vi "Create solenoid.vi"(7 "Variant":variant, 8 "error in (no error)":errorcluster, 9 "Reverse solenoid channel":string, 10 "Forward solenoid channel":string, 11 "Solenoids in":refnum<class "Solenoids.lvclass">) -> (0 "error out":errorcluster, 3 "Solenoids out":refnum<class "Solenoids.lvclass">)   [LabVIEW 2018, in "Pneumatics control.lvlib" / "Pneumatics.lvclass"]
doc: "This VI reads the string keys of the solenoid and sets them to the object using its Begin.vi"
uses:
  Pneumatics.lvclass
  Solenoids/Solenoids.lvclass
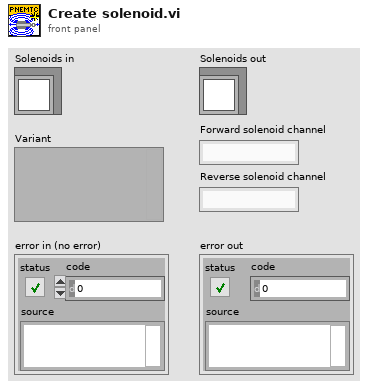
[diagram p1: front panel]
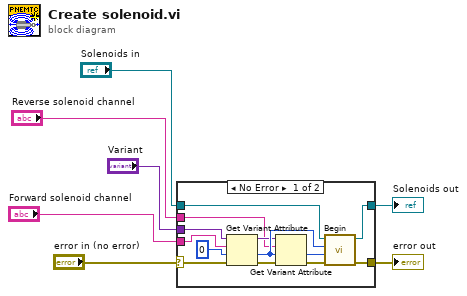
[diagram p0: block diagram]
diagram:
  n1 = case shown="No Error" "error in (no error)" {
    selector: "error in (no error)" -> [w12 w22]
    tunnel: [w19 w22] -> w7
    tunnel: "Variant" -> [w16 _]
    tunnel: "Solenoids in" -> [w11 w21]
    tunnel: [w10 w21] -> w3
    tunnel: "Forward solenoid channel" -> [w9 _]
    tunnel: "Reverse solenoid channel" -> [w8 _]
    frame No Error {
      n2 = Get Variant Attribute(Variant=w16, name=w9, default value (empty Variant)=u8 0, error in=w12) -> (duplicate Variant=w15:variant, value=w20:u8, error out=w13:errorcluster)  [unwired: 1 out]
      n3 = Get Variant Attribute(Variant=w15, name=w8, default value (empty Variant)=w20, error in=w13) -> (value=w18:u8, error out=w14:errorcluster)  [unwired: 2 out]
      n4 = call-dynamic "Begin.vi"("error in (no error)"=w14, "Reverse solenoid channel"=w18, "Forward Solenoid Channel"=w20, "Solenoids in"=w11) -> ("error out"=w19:errorcluster, "Solenoids out"=w10:refnum<class "Solenoids.lvclass">)  [unwired: 6 in]
    }
    frame Error {
    }
  }
  "error out" <- w7
  "Solenoids out" <- w3
